vi "min(a,b).vi"(9 "b":u8, 11 "a":u8) -> (2 "Out":u8)   [LabVIEW 2014]
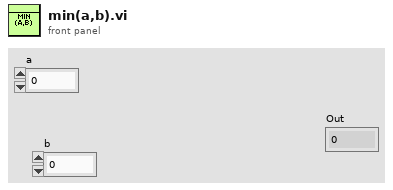
[diagram p1: front panel]
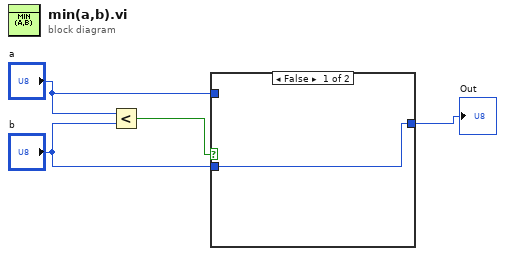
[diagram p0: block diagram]
diagram:
  n1 = Less?(x="a", y="b") -> (x < y?=w4:bool)
  n2 = case shown="False" w4 {
    tunnel: [w5 w6] -> w3
    tunnel: "a" -> [_ w6]
    tunnel: "b" -> [w5 _]
    frame False {
    }
    frame True {
    }
  }
  "Out" <- w3
